vi "checkError_2.vi"(7 "ID_EQUIPO":i32, 10 "code_IN":i32, 11 "Gen_IN":string="Generador 4") -> ()   [LabVIEW 2018]
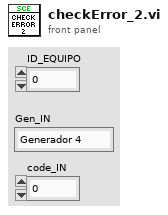
[diagram p1: front panel]
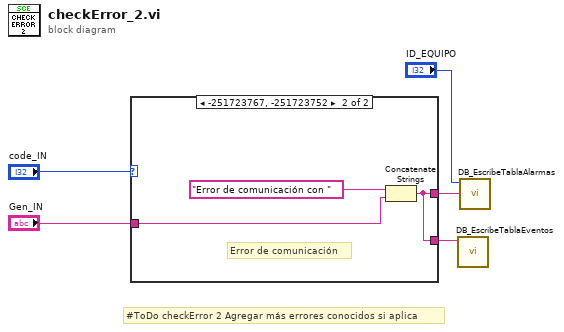
[diagram p0: block diagram]
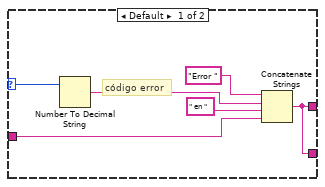
[diagram p2: hidden frame]
diagram:
  # "#ToDo checkError 2 Agregar más errores conocidos si aplica"
  n1 = case shown="-251723767, -251723752" "code_IN" {
    selector: "code_IN" -> [w9 _]
    tunnel: [w6 w14] -> w5
    tunnel: [w6 w14] -> w4
    tunnel: "Gen_IN" -> [w8 w12]
    frame Default {
      # "código error"
      n2 = Number To Decimal String(number=w9) -> (decimal integer string=w7:string)  [unwired: 1 in]
      n3 = Concatenate Strings("Error " ("string"), w7, " en " ("string"), w8) -> (w6:string)
    }
    frame -251723767, -251723752 {
      # "Error de comunicación"
      n4 = Concatenate Strings("Error de comunicación con " ("string"), w12) -> (w14:string)
    }
  }
  n5 = call "DB_EscribeTablaEventos.vi"("DESCRIPCION"=w4) -> ()  [unwired: 10 in, 1 out]
  n6 = call "DB_EscribeTablaAlarmas.vi"("MOTIVO"=w5, "ID_EQUIPO"="ID_EQUIPO") -> ()  [unwired: 9 in, 1 out]
